vi "Write Measured_Table_Ref.vi"(8 "error in (no error)":errorcluster, 10 "Measured_Table_Ref":refnum<vi>, 11 "DAQ970 in":refnum<class "DAQ970.lvclass">) -> (0 "error out":errorcluster, 3 "DAQ970 out":refnum<class "DAQ970.lvclass">)   [LabVIEW 2019, in "DAQ970.lvlib" / "DAQ970.lvclass"]
uses:
  Library/DAQ970.lvclass
  Library/DAQ970.lvclass/DAQ970.ctl
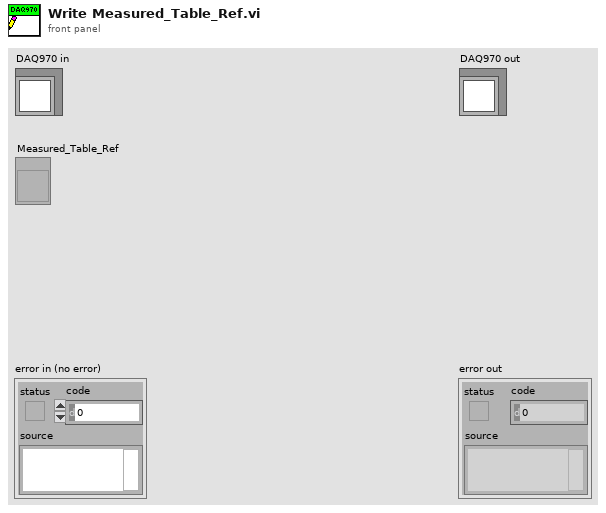
[diagram p1: front panel]
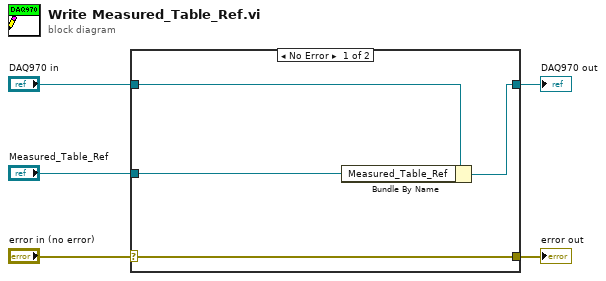
[diagram p0: block diagram]
diagram:
  n1 = case shown="No Error" "error in (no error)" {
    selector: "error in (no error)" -> [w9 w10]
    tunnel: [w9 w10] -> w4
    tunnel: [w7 w11] -> w2
    tunnel: "DAQ970 in" -> [w8 w11]
    tunnel: "Measured_Table_Ref" -> [w6 _]
    frame No Error {
      n2 = Bundle By Name(cluster=w8, "Measured_Table_Ref"=w6) -> (w7:refnum<class "DAQ970.lvclass">)
    }
    frame Error {
    }
  }
  "error out" <- w4
  "DAQ970 out" <- w2
